vi "Set Mode.vi"(6 "Mode":T1=enum."Tx", 8 "error in (no error)":errorcluster, 11 "TCPIP Communications in":refnum<class "TCPIP Communications.lvclass">) -> (0 "error out":errorcluster, 3 "TCPIP Communications out":refnum<class "TCPIP Communications.lvclass">)   [LabVIEW 2015, in "TCPIP Communications Framework.lvlib" / "TCPIP Communications.lvclass"]
uses:
  TCPIP Communications.lvclass
  Controls/Mode Select.ctl
  TCPIP Communications.lvclass/TCPIP Communications.ctl
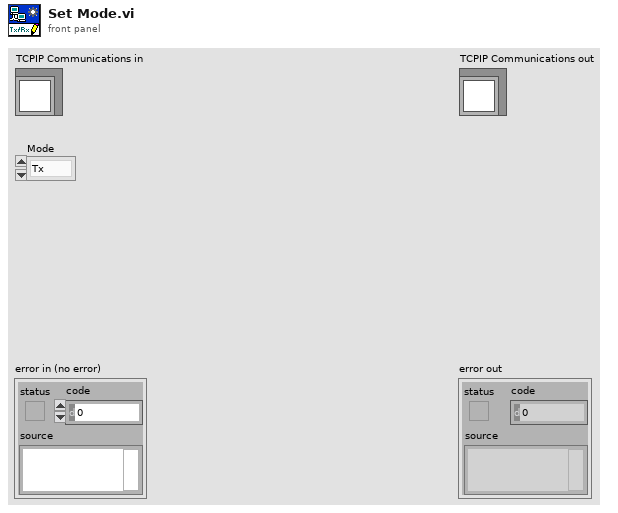
[diagram p1: front panel]
types:
  T1 = typedef "TCPIP Communications Framework.lvlib/TCPIP Communications.lvclass/Mode Select.ctl" = enum16{"Tx/Rx", "Tx", "Rx"}
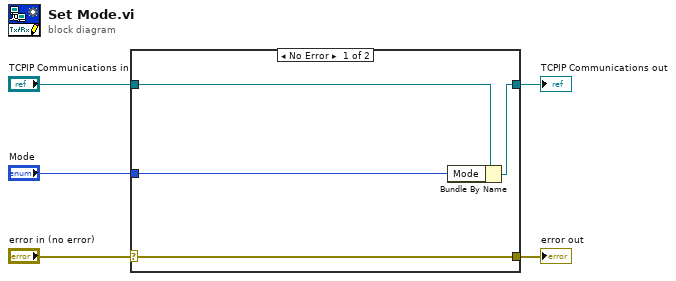
[diagram p0: block diagram]
diagram:
  n1 = case shown="No Error" "error in (no error)" {
    selector: "error in (no error)" -> [w9 w10]
    tunnel: [w9 w10] -> w4
    tunnel: [w7 w11] -> w2
    tunnel: "TCPIP Communications in" -> [w8 w11]
    tunnel: "Mode" -> [w6 _]
    frame No Error {
      n2 = Bundle By Name(cluster=w8, "Mode"=w6) -> (w7:refnum<class "TCPIP Communications.lvclass">)
    }
    frame Error {
    }
  }
  "error out" <- w4
  "TCPIP Communications out" <- w2
